vi "TLA_Execute.vi"(8 "error in (no error)":errorcluster caption="错误输入（无错误）", 9 "sqlParam":refnum<k24>[](array[refnum]), 10 "SQLstring":string, 11 "Traceability 引用句柄":refnum<k24>) -> (0 "error out":errorcluster caption="错误输出", 1 "sqlParam 2":refnum<k24>[](array[refnum]), 2 "TLA_ExecuteSQL":bool, 3 "Traceability 引用句柄输出":refnum<k24>)   [LabVIEW 2014, in "Traceability.lvlib"]
uses:
  D:/webservice/Traceability.dll
  Traceability.dll
  Traceability.lvlib
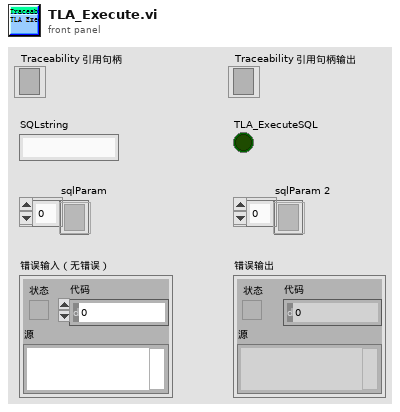
[diagram p1: front panel]
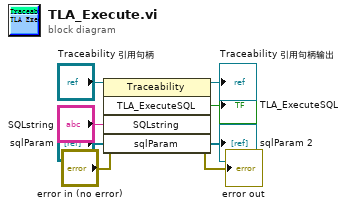
[diagram p0: block diagram]
diagram:
  n1 = invoke class="Traceability" method="TLA_ExecuteSQL"(reference="Traceability 引用句柄", error in="error in (no error)", "SQLstring"="SQLstring", "sqlParam"="sqlParam") -> (reference out=→"Traceability 引用句柄输出":refnum<k24>, error out=→"error out":errorcluster, "TLA_ExecuteSQL"=→"TLA_ExecuteSQL":bool, "sqlParam"=→"sqlParam 2":refnum<k24>[])  [unwired: 1 in, 1 out]
